vi "read response queue.vi"(11 "communicator message in":refnum<class "communicator message.lvclass">) -> (2 "communicator":refnum<class "communicator.lvclass">, 3 "communicator message out":refnum<class "communicator message.lvclass">)   [LabVIEW 2015, in "communicator message.lvclass"]
uses:
  communicator message.lvclass
  communicator/communicator.lvclass
  communicator message.lvclass/communicator message.ctl
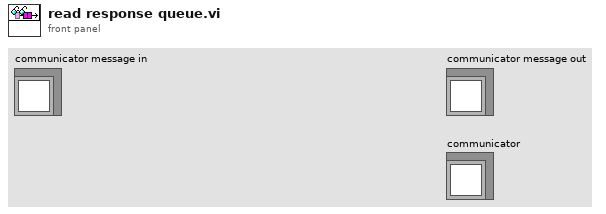
[diagram p1: front panel]
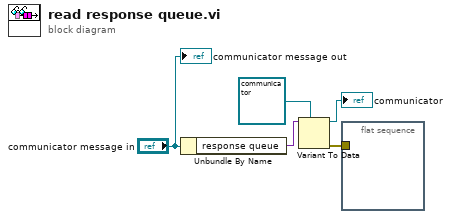
[diagram p0: block diagram]
diagram:
  n1 = Unbundle By Name("communicator message in") -> ("response queue"=w4:variant)
  n2 = Variant To Data(type=refnum<class "communicator.lvclass"> refnum ("communicator"), Variant=w4) -> (data=→"communicator":refnum<class "communicator.lvclass">, error out=w1:errorcluster)  [unwired: 1 in]
  n3 = flat-sequence {
    tunnel: w1 -> [_]
    frame #0 {
    }
  }
  "communicator message out" <- "communicator message in"
